vi "Ist-Zustand Position.vi"(8 "Fehler (Eingang, kein Fehler)":errorcluster, 10 "TPDO2 object in":refnum<k20>, 11 "TPDO1 object in":refnum<k20>) -> (0 "error out":errorcluster, 3 "Ist-Zustand Position":cluster{"Position":dbl, "Geschwindigkeit":dbl})   [LabVIEW 2014]
uses:
  <vilib>/CANopenLib/CANOPEN.llb/CANopen Fetch from Data [I32].vi
  <vilib>/CANopenLib/CANOPEN.llb/CANopen Fetch from Data [U16].vi
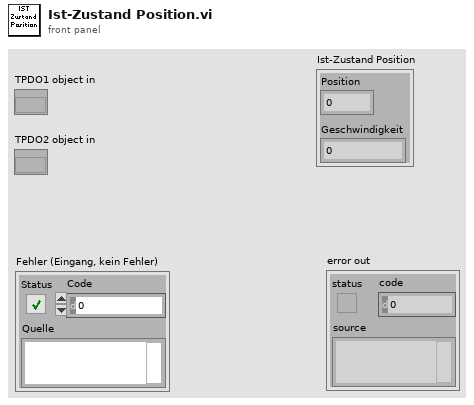
[diagram p1: front panel]
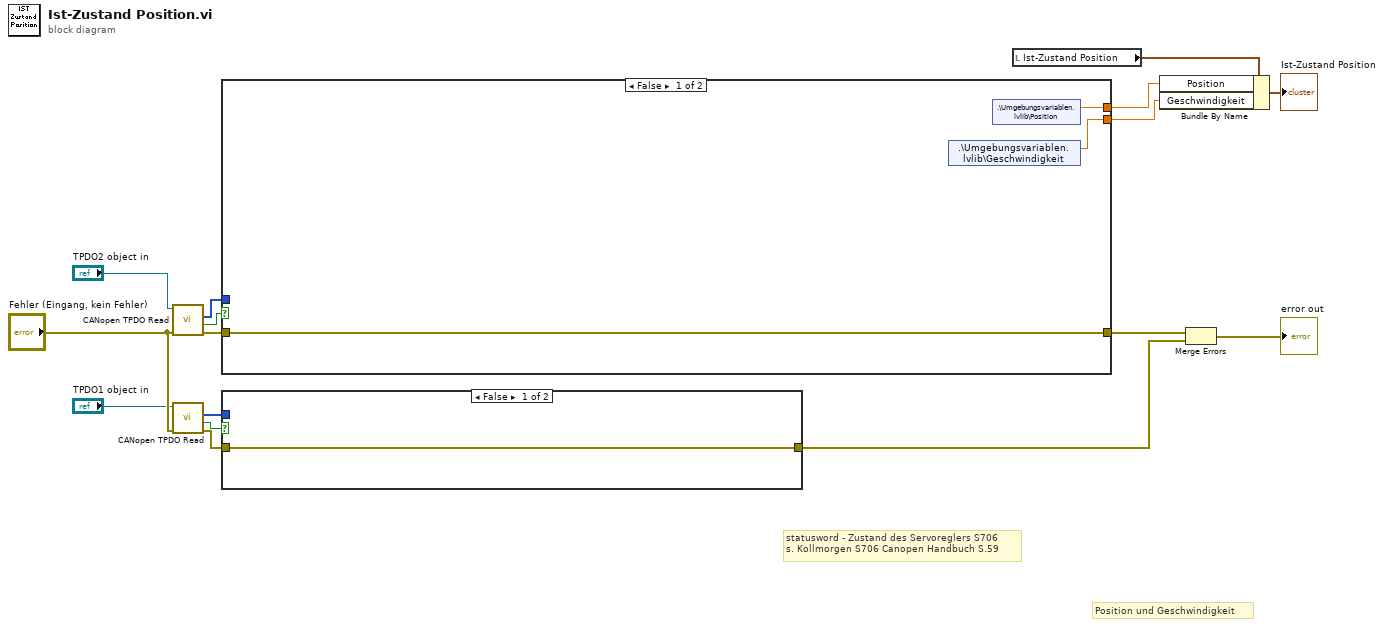
[diagram p0: block diagram]
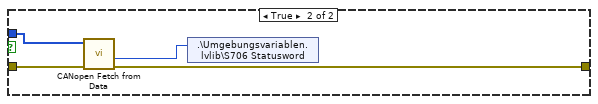
[diagram p2: hidden frame]
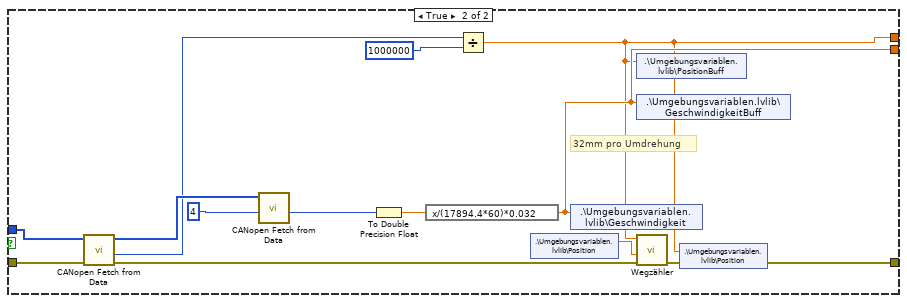
[diagram p3: hidden frame]
diagram:
  # "Position und Geschwindigkeit"
  # "statusword - Zustand des Servoreglers S706\ns. Kollmorgen S706 Canopen Handbuch S.59"
  n1 = call <vilib>:"CANopen TPDO Read.vi"("error in (no error)"="Fehler (Eingang, kein Fehler)", "TPDO object in"="TPDO2 object in") -> ("error out"=w13:errorcluster, "new data?"=w15:bool, "data"=w14:u8[])  [unwired: 5 in, 2 out]
  n2 = call <vilib>:"CANopen TPDO Read.vi"("error in (no error)"="Fehler (Eingang, kein Fehler)", "TPDO object in"="TPDO1 object in") -> ("error out"=w4:errorcluster, "new data?"=w7:bool, "data"=w5:u8[])  [unwired: 5 in, 2 out]
  n3 = case shown="False" w15 {
    tunnel: w14 -> [_ w33]
    tunnel: w13 -> [w19 w29]
    tunnel: [w19 w20] -> w2
    tunnel: [w18 w22] -> w10
    tunnel: [w17 w23] -> w9
    frame False {
      n4 = shared-variable ".\\Umgebungsvariablen.lvlib\\Geschwindigkeit"() -> (w17:dbl)  [unwired: 1 in, 1 out]
      n5 = shared-variable ".\\Umgebungsvariablen.lvlib\\Position"() -> (w18:dbl)  [unwired: 1 in, 1 out]
    }
    frame True {
      # "32mm pro Umdrehung"
      n6 = call-poly <vilib>:"CANopen Fetch from Data.vi"("error in (no error)"=w29, "CANopen data in"=w33) -> ("error out"=w28:errorcluster, "signed 32-bit integer"=w27:i32, "CANopen data out"=w32:u8[])  [unwired: 7 in]
      n7 = call-poly <vilib>:"CANopen Fetch from Data.vi"("offset (0)"=u32 4, "CANopen data in"=w32) -> ("signed 32-bit integer"=w25:i32)  [unwired: 7 in, 2 out]
      n8 = To Double Precision Float(number=w25) -> (double precision float=w24:dbl)
      n9 = expression code="x/(17894.4*60)*0.032"(w24) -> (w23:dbl)
      n10 = Divide(x=w27, y=1000000) -> (x/y=w22:dbl)
      n11 = shared-variable ".\\Umgebungsvariablen.lvlib\\Position"() -> (w30:dbl)  [unwired: 1 in, 1 out]
      n12 = shared-variable ".\\Umgebungsvariablen.lvlib\\Geschwindigkeit"(w23) -> ()  [unwired: 1 in, 1 out]
      n13 = shared-variable ".\\Umgebungsvariablen.lvlib\\PositionBuff"(w22) -> ()  [unwired: 1 in, 1 out]
      n14 = shared-variable ".\\Umgebungsvariablen.lvlib\\GeschwindigkeitBuff"(w23) -> ()  [unwired: 1 in, 1 out]
      n15 = call "Wegzähler.vi"("error in (no error)"=w28, "letzter Wert"=w30, "aktueller Wert"=w22) -> ("error out"=w21:errorcluster)  [unwired: 8 in]
      n16 = shared-variable ".\\Umgebungsvariablen.lvlib\\Position"(w22, error in=w21) -> (error out=w20:errorcluster)
    }
  }
  n17 = case shown="False" w7 {
    tunnel: w5 -> [_ w38]
    tunnel: w4 -> [w34 w37]
    tunnel: [w34 w36] -> w3
    frame False {
    }
    frame True {
      n18 = call-poly <vilib>:"CANopen Fetch from Data.vi"("error in (no error)"=w37, "CANopen data in"=w38) -> ("error out"=w36:errorcluster, "unsigned 16-bit integer"=w35:u16)  [unwired: 7 in, 1 out]
      n19 = shared-variable ".\\Umgebungsvariablen.lvlib\\S706 Statusword"(w35) -> ()  [unwired: 1 in, 1 out]
    }
  }
  n20 = local read "Ist-Zustand Position"() -> (w12:cluster{"Position":dbl, "Geschwindigkeit":dbl})
  n21 = Bundle By Name(cluster=w12, "Position"=w10, "Geschwindigkeit"=w9) -> (→"Ist-Zustand Position":cluster{"Position":dbl, "Geschwindigkeit":dbl})
  n22 = Merge Errors(w2, w3) -> (→"error out":errorcluster)
